vi "Parse Array.vi"(8 "Error In":errorcluster, 11 "Array XML String Input":string) -> (0 "Error Out":errorcluster, 2 "Rest String":string, 3 "Array Val":string)   [LabVIEW 2017, in "MU_3SL_interface.lvlib"]
uses:
  MU_3SL_interface.lvlib
  <vilib>/regexp/Match Regular Expression.xnode
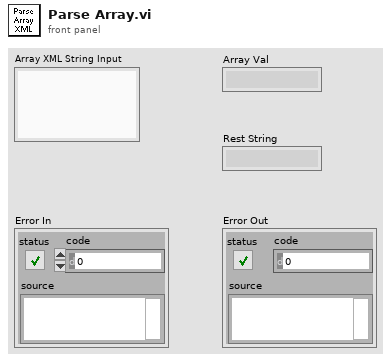
[diagram p1: front panel]
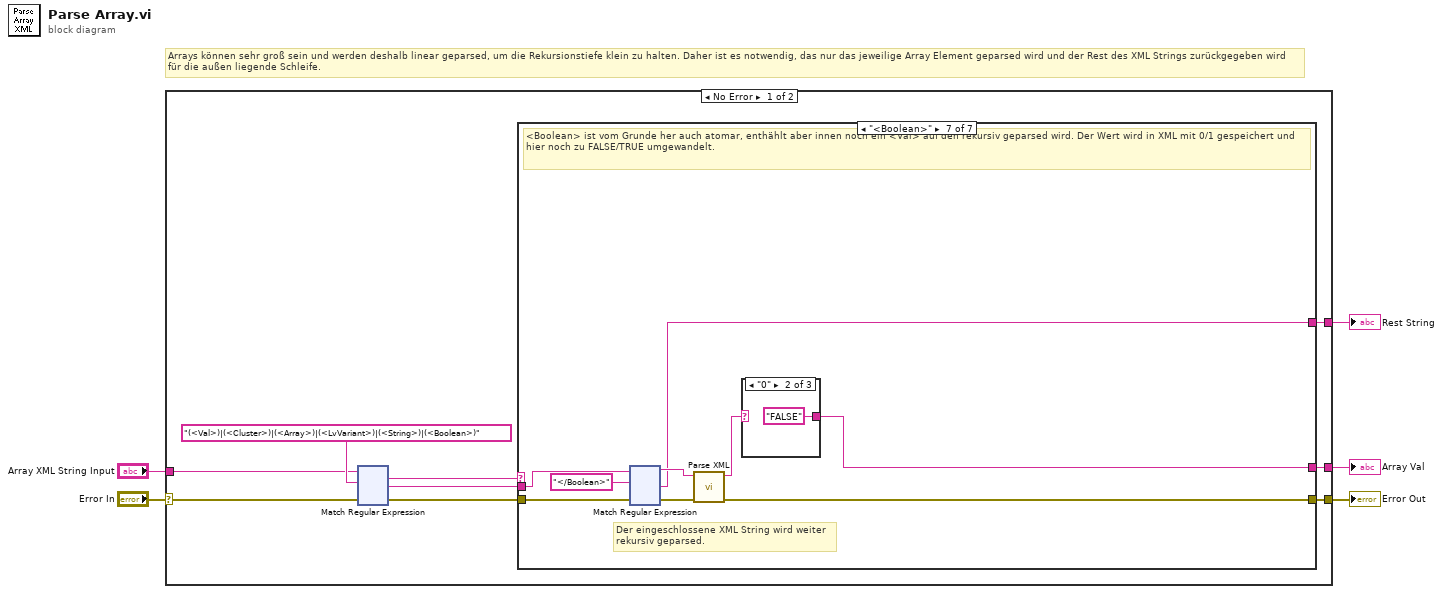
[diagram p0: block diagram]
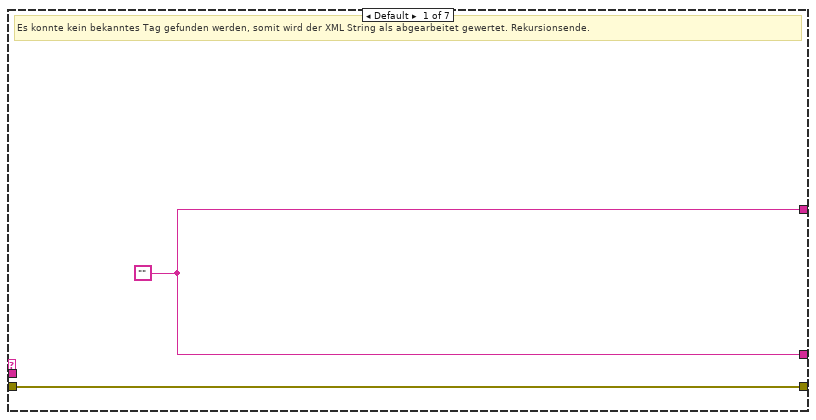
[diagram p2: hidden frame]
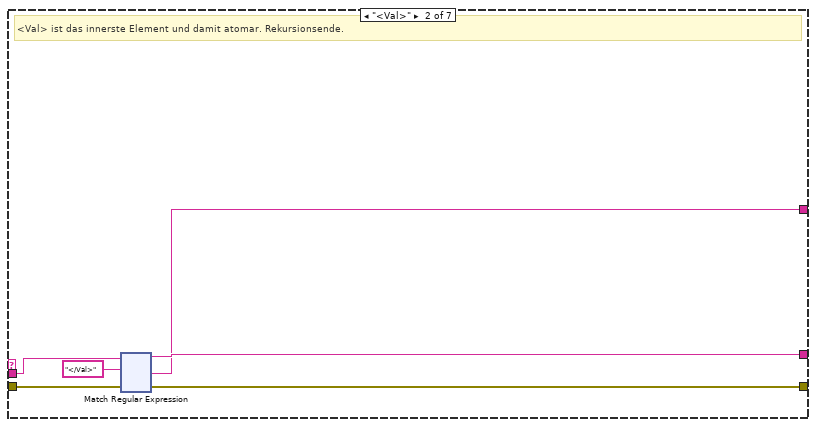
[diagram p3: hidden frame]
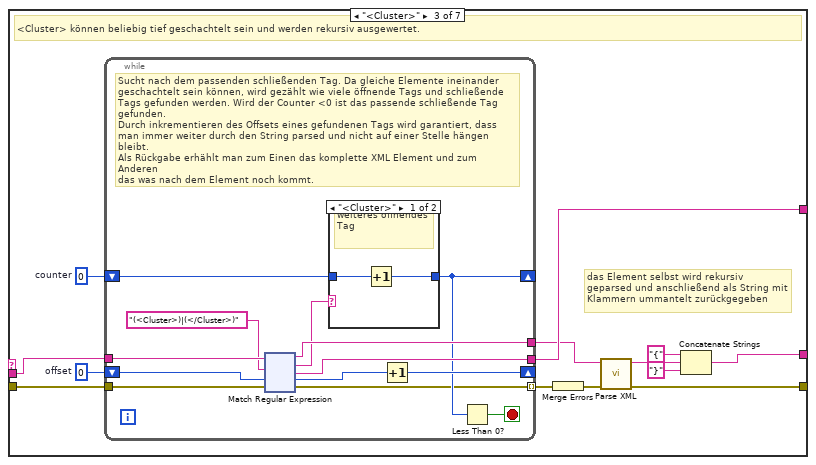
[diagram p4: hidden frame]
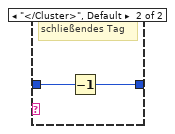
[diagram p5: hidden frame]
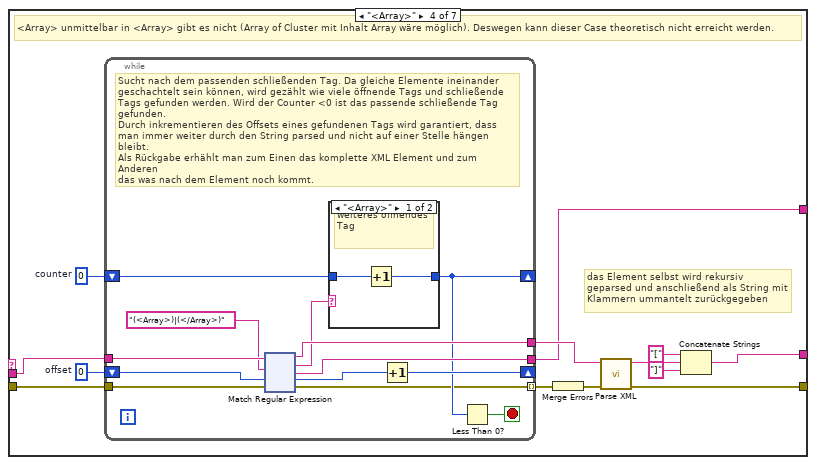
[diagram p6: hidden frame]
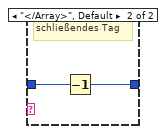
[diagram p7: hidden frame]
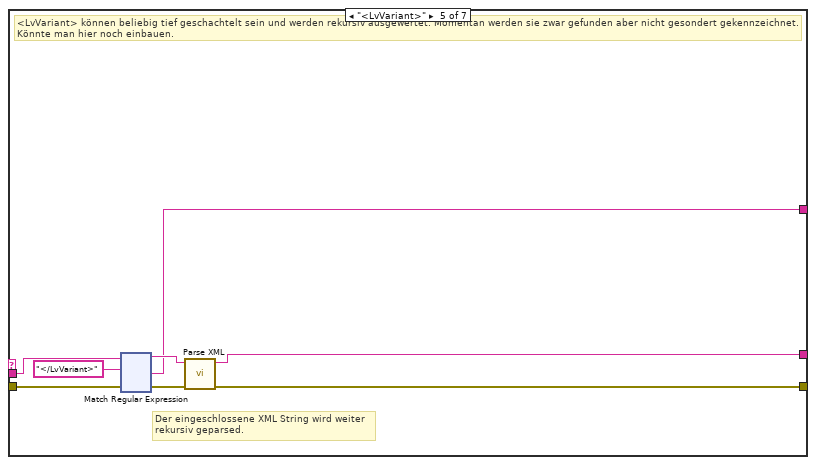
[diagram p8: hidden frame]
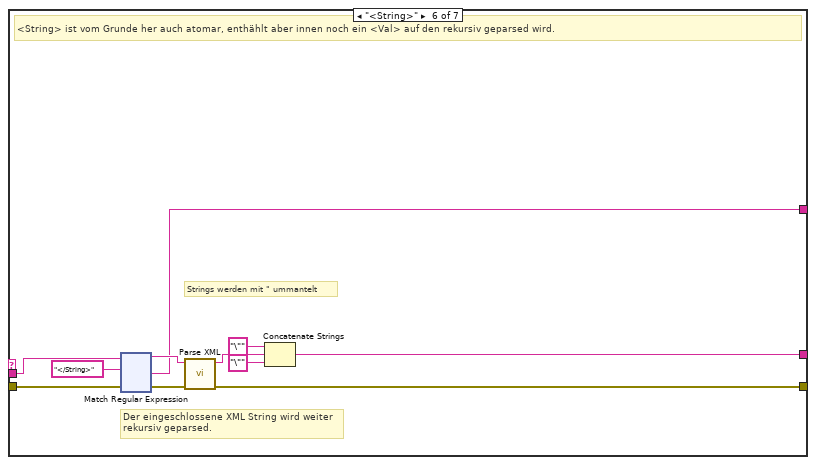
[diagram p9: hidden frame]
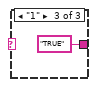
[diagram p11: hidden frame]
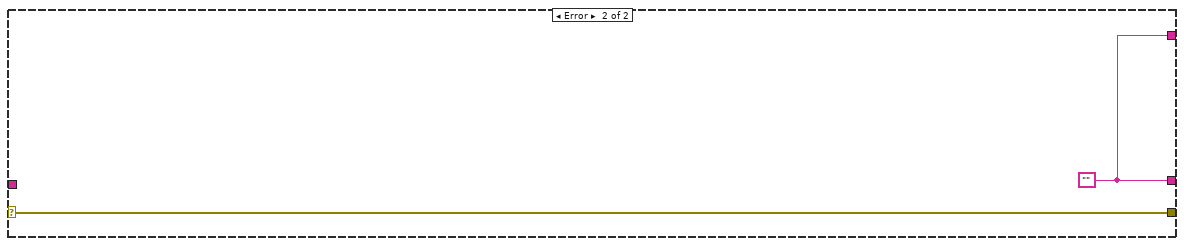
[diagram p12: hidden frame]
diagram:
  # "Arrays können sehr groß sein und werden deshalb linear geparsed, um die Rekursionstiefe klein zu halten. Daher ist es notwendig, das nur das jeweilige Array Element geparsed wird und der Rest des XML Strings zurückgegeben wird\nfür die außen liegende Schleife."
  n1 = case shown="No Error" "Error In" {
    selector: "Error In" -> [w8 w913]
    tunnel: "Array XML String Input" -> [w13 _]
    tunnel: [w10 w912] -> w4
    tunnel: [w9 w912] -> w3
    tunnel: [w6 w913] -> w1
    frame No Error {
      n2 = xnode "Match Regular Expression"("input string"=w13, "regular expression"="(<Val>)|(<Cluster>)|(<Array>)|(<LvVariant>)|(<String>)|(<Boolean>)", "error in"=w8) -> ("whole match"=w12:string, "after match"=w11:string, "error out"=w7:errorcluster)  [unwired: 3 in, 2 out]
      n3 = case shown="\"<Boolean>\"" w12 {
        tunnel: w11 -> [_ w21 w149 w293 w431 w556 w679]
        tunnel: [w16 w20 w147 w285 w429 w551 w676] -> w10
        tunnel: [w16 w19 w148 w286 w428 w550 w675] -> w9
        tunnel: w7 -> [w15 w18 w146 w284 w427 w549 w674]
        tunnel: [w15 w17 w145 w281 w425 w547 w672] -> w6
        frame Default {
          w16 = ""
          # "Es konnte kein bekanntes Tag gefunden werden, somit wird der XML String als abgearbeitet gewertet. Rekursionsende."
        }
        frame "<Val>" {
          # "<Val> ist das innerste Element und damit atomar. Rekursionsende."
          n4 = xnode "Match Regular Expression"("input string"=w21, "regular expression"="</Val>", "error in"=w18) -> ("before match"=w20:string, "after match"=w19:string, "error out"=w17:errorcluster)  [unwired: 3 in, 2 out]
        }
        frame "<Cluster>" {
          w140 = 0  # offset
          w141 = 0  # counter
          # "das Element selbst wird rekursiv geparsed und anschließend als String mit Klammern ummantelt zurückgegeben"
          # "<Cluster> können beliebig tief geschachtelt sein und werden rekursiv ausgewertet."
          n5 = while {
            tunnel: [w159] -> w148
            shift-right: [w155] -> _
            shift-left: w140 -> [w157]
            shift-right: [w153] -> _
            shift-left: w141 -> [w154]
            tunnel: w149 -> [w162]
            tunnel: [w160] -> w144
            tunnel: w146 -> [w151]
            tunnel: [w150] -> w138 mode=indexing
            stop <- w152 stop-if-true
            # "Sucht nach dem passenden schließenden Tag. Da gleiche Elemente ineinander\ngeschachtelt sein können, wird gezählt wie viele öffnende Tags und schließende\nTags gefunden werden. Wird der Counter <0 ist das passende schließende Tag\ngefunden.\nDurch inkrementieren des Offsets eines gefundenen Tags wird garantiert, dass \nman immer weiter durch den String parsed und nicht auf einer Stelle hängen bleibt.\nAls Rückgabe erhählt man zum Einen das komplette XML Element und zum Anderen\ndas was nach dem Element noch kommt."
            n6 = xnode "Match Regular Expression"("input string"=w162, "regular expression"="(<Cluster>)|(</Cluster>)", "offset (0)"=w157, "error in"=w151) -> ("before match"=w160:string, "whole match"=w158:string, "after match"=w159:string, "offset past match"=w156:i32, "error out"=w150:errorcluster)  [unwired: 2 in]
            n7 = case shown="\"<Cluster>\"" w158 {
              tunnel: w154 -> [w164 w166]
              tunnel: [w163 w165] -> w153
              frame "<Cluster>" {
                # "weiteres öffnendes Tag"
                n8 = Increment(x=w164) -> (x+1=w163:i32)
              }
              frame "</Cluster>", Default {
                # "schließendes Tag"
                n9 = Decrement(x=w166) -> (x-1=w165:i32)
              }
            }
            n10 = Increment(x=w156) -> (x+1=w155:i32)
            n11 = Less Than 0?(x=w153) -> (x < 0?=w152:bool)
          }
          n12 = Merge Errors(w138) -> (w137:errorcluster)
          n13 = call "Parse XML.vi"("Error In"=w137, "XML String Input"=w144) -> ("Error Out"=w145:errorcluster, "Parsed Value"=w139:string)  [unwired: 8 in]
          n14 = Concatenate Strings("{" ("string"), w139, "}" ("string")) -> (w147:string)
        }
        frame "<Array>" {
          w288 = 0  # offset
          w289 = 0  # counter
          # "das Element selbst wird rekursiv geparsed und anschließend als String mit Klammern ummantelt zurückgegeben"
          # "<Array> unmittelbar in <Array> gibt es nicht (Array of Cluster mit Inhalt Array wäre möglich). Deswegen kann dieser Case theoretisch nicht erreicht werden."
          n15 = while {
            tunnel: [w303] -> w286
            shift-right: [w299] -> _
            shift-left: w288 -> [w301]
            shift-right: [w297] -> _
            shift-left: w289 -> [w298]
            tunnel: w293 -> [w306]
            tunnel: [w304] -> w292
            tunnel: w284 -> [w295]
            tunnel: [w294] -> w283 mode=indexing
            stop <- w296 stop-if-true
            # "Sucht nach dem passenden schließenden Tag. Da gleiche Elemente ineinander\ngeschachtelt sein können, wird gezählt wie viele öffnende Tags und schließende\nTags gefunden werden. Wird der Counter <0 ist das passende schließende Tag\ngefunden.\nDurch inkrementieren des Offsets eines gefundenen Tags wird garantiert, dass \nman immer weiter durch den String parsed und nicht auf einer Stelle hängen bleibt.\nAls Rückgabe erhählt man zum Einen das komplette XML Element und zum Anderen\ndas was nach dem Element noch kommt."
            n16 = xnode "Match Regular Expression"("input string"=w306, "regular expression"="(<Array>)|(</Array>)", "offset (0)"=w301, "error in"=w295) -> ("before match"=w304:string, "whole match"=w302:string, "after match"=w303:string, "offset past match"=w300:i32, "error out"=w294:errorcluster)  [unwired: 2 in]
            n17 = case shown="\"<Array>\"" w302 {
              tunnel: w298 -> [w308 w310]
              tunnel: [w307 w309] -> w297
              frame "<Array>" {
                # "weiteres öffnendes Tag"
                n18 = Increment(x=w308) -> (x+1=w307:i32)
              }
              frame "</Array>", Default {
                # "schließendes Tag"
                n19 = Decrement(x=w310) -> (x-1=w309:i32)
              }
            }
            n20 = Increment(x=w300) -> (x+1=w299:i32)
            n21 = Less Than 0?(x=w297) -> (x < 0?=w296:bool)
          }
          n22 = Merge Errors(w283) -> (w282:errorcluster)
          n23 = call "Parse XML.vi"("Error In"=w282, "XML String Input"=w292) -> ("Error Out"=w281:errorcluster, "Parsed Value"=w287:string)  [unwired: 8 in]
          n24 = Concatenate Strings("[" ("string"), w287, "]" ("string")) -> (w285:string)
        }
        frame "<LvVariant>" {
          # "Der eingeschlossene XML String wird weiter \nrekursiv geparsed."
          # "<LvVariant> können beliebig tief geschachtelt sein und werden rekursiv ausgewertet. Momentan werden sie zwar gefunden aber nicht gesondert gekennzeichnet. Könnte man hier noch einbauen."
          n25 = xnode "Match Regular Expression"("input string"=w431, "regular expression"="</LvVariant>", "error in"=w427) -> ("before match"=w432:string, "after match"=w428:string, "error out"=w426:errorcluster)  [unwired: 3 in, 2 out]
          n26 = call "Parse XML.vi"("Error In"=w426, "XML String Input"=w432) -> ("Error Out"=w425:errorcluster, "Parsed Value"=w429:string)  [unwired: 8 in]
        }
        frame "<String>" {
          # "Strings werden mit \" ummantelt"
          # "Der eingeschlossene XML String wird weiter \nrekursiv geparsed."
          # "<String> ist vom Grunde her auch atomar, enthählt aber innen noch ein <Val> auf den rekursiv geparsed wird."
          n27 = xnode "Match Regular Expression"("input string"=w556, "regular expression"="</String>", "error in"=w549) -> ("before match"=w557:string, "after match"=w550:string, "error out"=w548:errorcluster)  [unwired: 3 in, 2 out]
          n28 = call "Parse XML.vi"("Error In"=w548, "XML String Input"=w557) -> ("Error Out"=w547:errorcluster, "Parsed Value"=w552:string)  [unwired: 8 in]
          n29 = Concatenate Strings("\"" ("string"), w552, "\"" ("string")) -> (w551:string)
        }
        frame "<Boolean>" {
          # "Der eingeschlossene XML String wird weiter \nrekursiv geparsed."
          # "<Boolean> ist vom Grunde her auch atomar, enthählt aber innen noch ein <Val> auf den rekursiv geparsed wird. Der Wert wird in XML mit 0/1 gespeichert und hier noch zu FALSE/TRUE umgewandelt."
          n30 = xnode "Match Regular Expression"("input string"=w679, "regular expression"="</Boolean>", "error in"=w674) -> ("before match"=w680:string, "after match"=w675:string, "error out"=w673:errorcluster)  [unwired: 3 in, 2 out]
          n31 = call "Parse XML.vi"("Error In"=w673, "XML String Input"=w680) -> ("Error Out"=w672:errorcluster, "Parsed Value"=w677:string)  [unwired: 8 in]
          n32 = case shown="\"0\"" w677 {
            selector: w677 -> [w681 _ _]
            tunnel: [w681 "FALSE" ("string") "TRUE" ("string")] -> w676
            frame Default {
            }
            frame "0" {
            }
            frame "1" {
            }
          }
        }
      }
    }
    frame Error {
      w912 = ""
    }
  }
  "Array Val" <- w4
  "Rest String" <- w3
  "Error Out" <- w1
